vi "Set Log Status.vi"(0 "status in":string, 11 "error in":errorcluster) -> (15 "error out":errorcluster)   [LabVIEW 2021, in "Converter Reusables.lvlib"]
uses:
  Converter Reusables.lvlib
  TypeDefs/Dictionary States.ctl
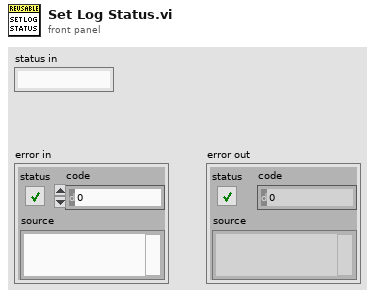
[diagram p1: front panel]
types:
  T1 = typedef "Converter Reusables.lvlib/Dictionary States.ctl" = enum16{"Set", "Get", "Delete", "Delete All"}
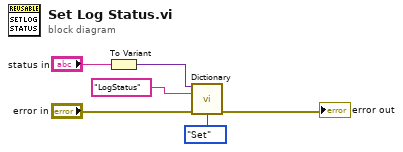
[diagram p0: block diagram]
diagram:
  n1 = To Variant(anything="status in") -> (Variant=w1:variant)
  n2 = call "Dictionary.vi"("variant in"=w1, "key"="LogStatus" ("Key"), "error in"="error in", "dict states"=Dictionary_States."Set" ("Dict States")) -> ("error out"=→"error out":errorcluster)  [unwired: 10 in, 1 out]
